vi "Read configuration.vi"(8 "error in":errorcluster, 11 "sbRIO-9651 in":refnum<class "sbRIO-9651.lvclass">) -> (0 "error out":errorcluster, 2 "configuration":refnum<class "NISE_CEF_serializable configuration.lvclass">, 3 "sbRIO-9651 out":refnum<class "sbRIO-9651.lvclass">)   [LabVIEW 2014, in "sbRIO-9651.lvclass"]
uses:
  sbRIO-9651.lvclass
  <vilib>/NI/Configuration Framework/serializable configuration/NISE_CEF_serializable configuration.lvclass
  <vilib>/NI/Configuration Framework/serializable node/NISE_CEF_serializable node.lvclass
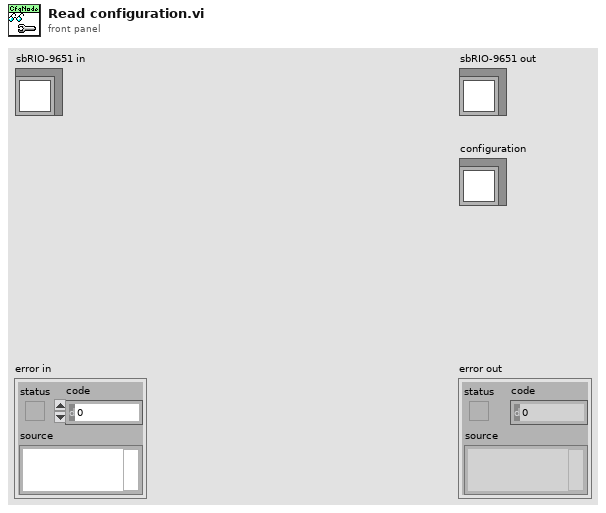
[diagram p1: front panel]
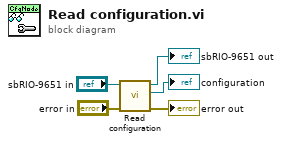
[diagram p0: block diagram]
diagram:
  n1 = call-parent "Read configuration.vi"("error in"="error in", "NISE_CEF_serializable node in"="sbRIO-9651 in") -> ("error out"=→"error out":errorcluster, "configuration"=→"configuration":refnum<class "NISE_CEF_serializable configuration.lvclass">, "NISE_CEF_serializable node out"=→"sbRIO-9651 out":refnum<class "sbRIO-9651.lvclass">)  [unwired: 7 in]
